vi "Zero.vi"() -> ()   [LabVIEW 2023, in "Anritsu.lvlib"]
uses:
  Anritsu.lvlib
panel:
  in  "VISA CMD":string="SYST:PRES"
  in  "VISA in":refnum<visa-resource-name>
  in  "error in":errorcluster
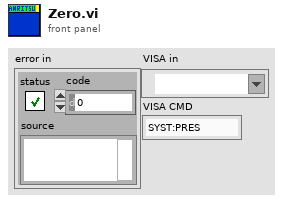
[diagram p1: front panel]
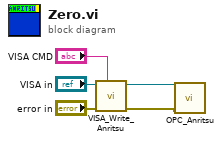
[diagram p0: block diagram]
diagram:
  n1 = call "VISA_Write_Anritsu.vi"("VISA CMD"="VISA CMD", "error in"="error in", "VISA in"="VISA in") -> ("error out"=w2:errorcluster, "VISA out"=w1:refnum<visa-resource-name>)  [unwired: 7 in]
  n2 = call "OPC_Anritsu.vi"("error in (no error)"=w2, "VISA resource name"=w1) -> ()  [unwired: 8 in, 2 out]
